vi "Create File Path.vi"(1 "Folder Path":path=path "c:/Temp/Data.lvm") -> (0 "File Path":path)   [LabVIEW 2019]
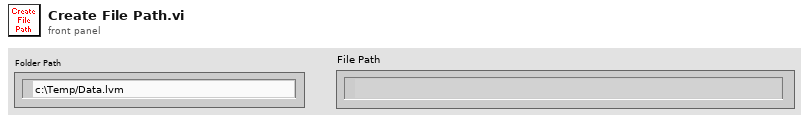
[diagram p1: front panel]
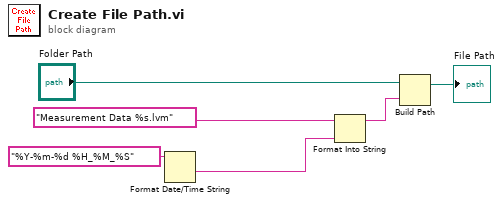
[diagram p0: block diagram]
diagram:
  n1 = Format Date/Time String(time format string (%c)="%Y-%m-%d %H_%M_%S") -> (date/time string=w1:string)  [unwired: 2 in]
  n2 = Format Into String(format string="Measurement Data %s.lvm", w1) -> (resulting string=w5:string)  [unwired: 2 in, 1 out]
  n3 = Build Path(base path="Folder Path", name or relative path=w5) -> (appended path=→"File Path":path)
